vi "Emballage_DefinirEntêtePiedpageImprimante.vi"(8 "Error in":errorcluster caption="Error in (no error)") -> (0 "Error out":errorcluster)   [LabVIEW 2020]
panel:
  out "standard output 2":string caption="sortie standard"
  out "standard error 2":string caption="erreur standard"
  out "standard error":string caption="erreur standard"
  out "standard output":string caption="sortie standard"
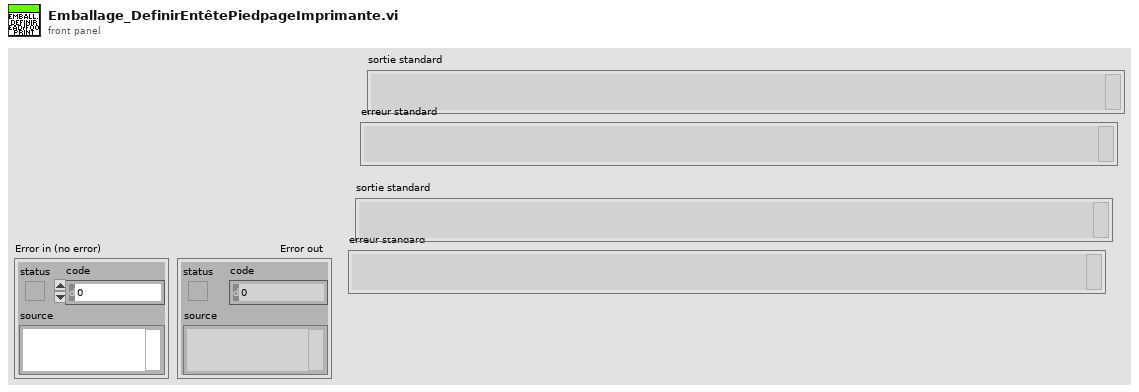
[diagram p1: front panel]
types:
  T1 = cluster{"header":string, "footer":string, "margin_bottom":string, "margin_left":string, "margin_right":string, "margin_top":string}
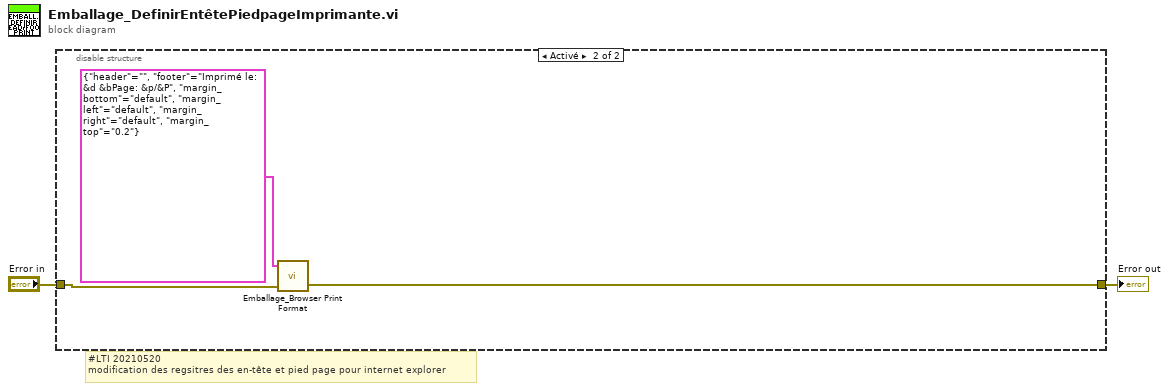
[diagram p0: block diagram]
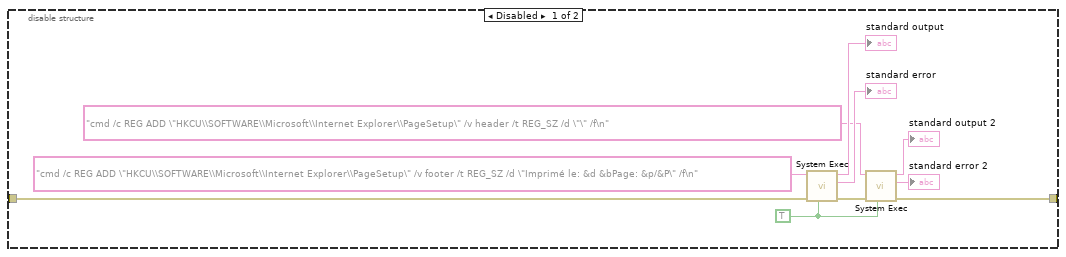
[diagram p2: hidden frame]
diagram:
  # "#LTI 20210520\nmodification des regsitres des en-tête et pied page pour internet explorer"
  n1 = disable-structure shown="Activé" {
    disable-tunnel: "Error in" -> [w10 w15]
    disable-tunnel: [w7 w14] -> w1
    frame Disabled {
      w3 = TRUE ("run minimized? (F)")
      n2 = call <vilib>:"System Exec.vi"("run minimized? (F)"=w3, "error in (no error)"=w10, "command line"="cmd /c REG ADD \"HKCU\\SOFTWARE\\Microsoft\\Internet Explorer\\PageSetup\" /v footer /t REG_SZ /d \"Imprimé le: &d &bPage: &p/&P\" /f\n") -> ("error out"=w8:errorcluster, "standard error"=→"standard error":string, "standard output"=→"standard output":string)  [unwired: 5 in, 1 out]
      n3 = call <vilib>:"System Exec.vi"("run minimized? (F)"=w3, "error in (no error)"=w8, "command line"="cmd /c REG ADD \"HKCU\\SOFTWARE\\Microsoft\\Internet Explorer\\PageSetup\" /v header /t REG_SZ /d \"\" /f\n") -> ("error out"=w7:errorcluster, "standard error"=→"standard error 2":string, "standard output"=→"standard output 2":string)  [unwired: 5 in, 1 out]
    }
    frame Enabled {
      n4 = call "Emballage_Browser Print Format.vi"("error in (no error)"=w15, "Format"=T1 {"header"="", "footer"="Imprimé le: &d &bPage: &p/&P", "margin_bottom"="default", "margin_left"="default", "margin_right"="default", "margin_top"="0.2"}) -> ("error out"=w14:errorcluster)  [unwired: 2 in, 1 out]
    }
  }
  "Error out" <- w1
